vi "get_status_modelocked.vi"(8 "error in (no error)":errorcluster, 11 "LightSourceMH110124MaiTai in":refnum<class "LightSourceMH110124MaiTai.lvclass">) -> (0 "error out":errorcluster, 1 "Emission":bool, 2 "Pulsing":bool, 3 "LightSourceMH110124MaiTai out":refnum<class "LightSourceMH110124MaiTai.lvclass">)   [LabVIEW 2010, in "LightSourceMH110124MaiTai.lvclass"]
uses:
  LightSourceMH110124MaiTai.lvclass
  LightSourceMH110124MaiTai.lvclass/LightSourceMH110124MaiTai.ctl
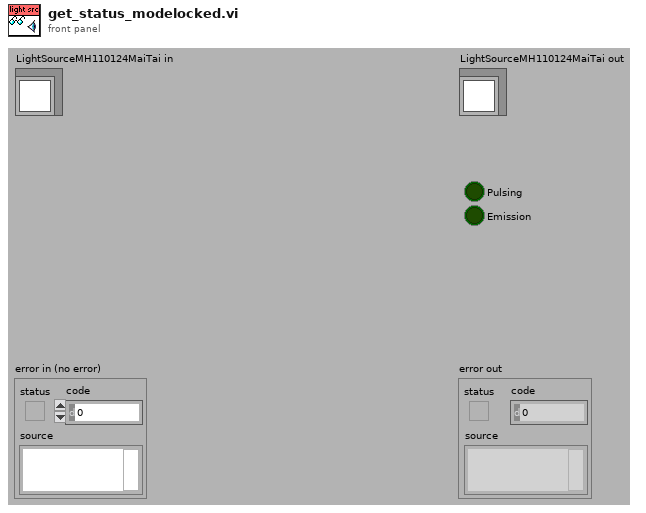
[diagram p1: front panel]
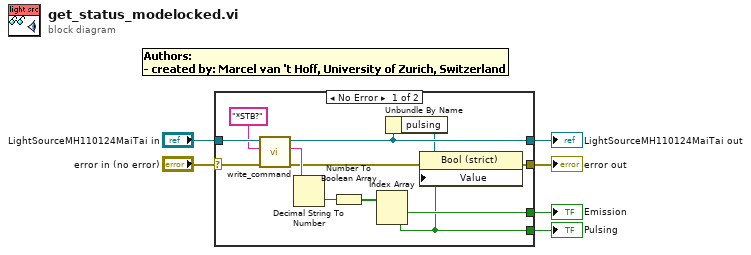
[diagram p0: block diagram]
diagram:
  n1 = case shown="No Error" "error in (no error)" {
    selector: "error in (no error)" -> [w17 w20]
    tunnel: [w9 w20] -> w1
    tunnel: [w11 w19] -> w3
    tunnel: "LightSourceMH110124MaiTai in" -> [w18 w19]
    tunnel: [w12 _] -> w5
    tunnel: [w7 _] -> w6
    frame No Error {
      n2 = call-dynamic "write_command.vi"("error in (no error)"=w17, "string to write"="*STB?", "LightSourceMH110124MaiTai in"=w18) -> ("error out"=w10:errorcluster, "read string"=w13:string, "LightSourceMH110124MaiTai out"=w11:refnum<class "LightSourceMH110124MaiTai.lvclass">)  [unwired: 6 in]
      n3 = Decimal String To Number(string=w13) -> (number=w15:i32)  [unwired: 2 in, 1 out]
      n4 = Number To Boolean Array(number=w15) -> (Boolean array=w14:bool[])
      n5 = Index Array(array=w14) -> (element #1=w12:bool, element #2=w7:bool)  [unwired: 2 in]
      n6 = Unbundle By Name(w11) -> ("pulsing"=w8:refnum<vi>)
      n7 = property class="Bool (strict)"(reference=w8, error in=w10, "Value"=w7) -> (error out=w9:errorcluster)  [unwired: 1 out]
    }
    frame Error {
    }
  }
  "error out" <- w1
  "LightSourceMH110124MaiTai out" <- w3
  "Emission" <- w5
  "Pulsing" <- w6
